vi "ClimbExecuteLogic.vi"(8 "error in (no error)":errorcluster, 9 "PullLS":bool, 10 "ReachLS":bool, 11 "SensorPosition":dbl) -> (0 "error out":errorcluster, 2 "ClimbStates":T1, 3 "MotorDemand":dbl)   [LabVIEW 2023]
doc: "Holds the \"insides\" for the elevator execution"
uses:
  <vilib>/Rock Robotics/WPI/ThirdParty/JAS_Junk/TrajLib/Trajectory_Library.lvlib
  ClimbGlobal.vi
  ClimbStates.ctl
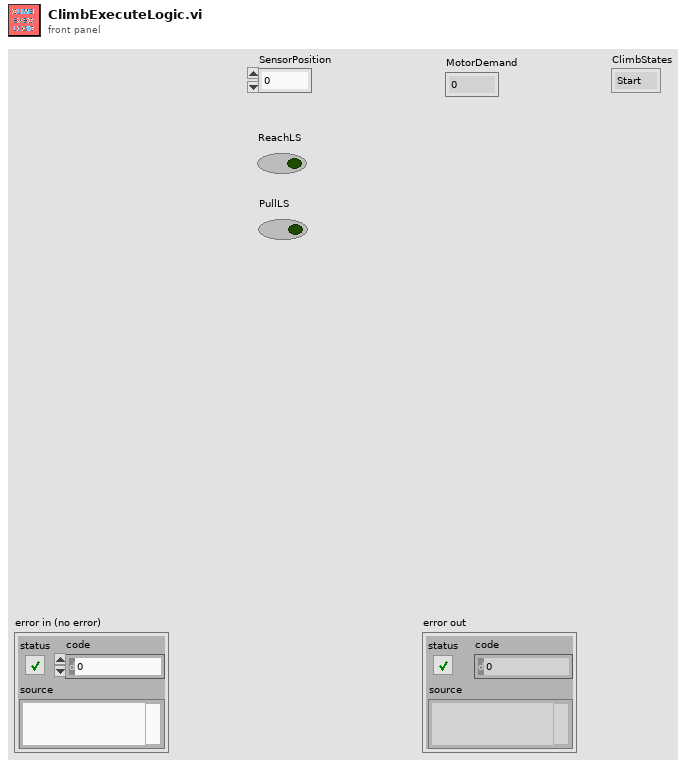
[diagram p1: front panel]
types:
  T1 = typedef "ClimbStates.ctl" = enum16{"Start", "WaitForCommands", "ClimbRest", "ClimbReach", "ClimbPull", "ClimbHang"}
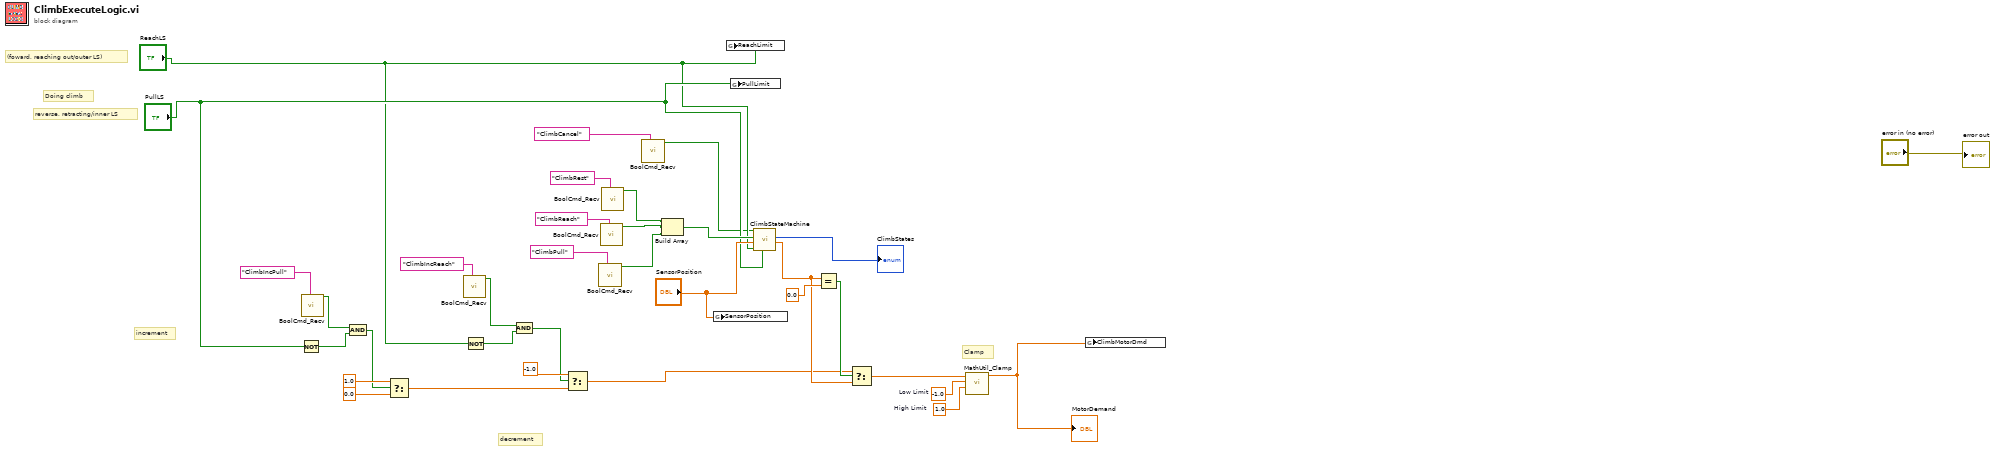
[diagram p0: block diagram]
diagram:
  w30 = 1.0  # High Limit
  w29 = -1.0  # Low Limit
  # "Doing climb"
  # "reverse, retracting/inner LS"
  # "(foward, reaching out/outer LS)"
  # "Clamp"
  # "increment"
  # "decrement"
  n1 = Not(x="PullLS") -> (.not. x?=w13:bool)
  n2 = call <vilib>:"BoolCmd_Recv.vi"("Command Name"="ClimbIncPull") -> ("New Request"=w1:bool)  [unwired: 9 in, 1 out]
  n3 = And(x=w1, y=w13) -> (x .and. y?=w12:bool)
  n4 = Select(t=1.0, s=w12, f=0.0) -> (s? t:f=w24:dbl)
  n5 = call <vilib>:"BoolCmd_Recv.vi"("Command Name"="ClimbIncReach") -> ("New Request"=w2:bool)  [unwired: 9 in, 1 out]
  n6 = Not(x="ReachLS") -> (.not. x?=w10:bool)
  n7 = And(x=w2, y=w10) -> (x .and. y?=w11:bool)
  n8 = Select(t=-1.0, s=w11, f=w24) -> (s? t:f=w22:dbl)
  n9 = call <vilib>:"BoolCmd_Recv.vi"("Command Name"="ClimbPull") -> ("New Request"=w3:bool)  [unwired: 9 in, 1 out]
  n10 = call <vilib>:"BoolCmd_Recv.vi"("Command Name"="ClimbReach") -> ("New Request"=w4:bool)  [unwired: 9 in, 1 out]
  n11 = call <vilib>:"BoolCmd_Recv.vi"("Command Name"="ClimbRest") -> ("New Request"=w5:bool)  [unwired: 9 in, 1 out]
  n12 = call <vilib>:"BoolCmd_Recv.vi"("Command Name"="ClimbCancel") -> ("New Request"=w6:bool)  [unwired: 9 in, 1 out]
  n13 = Build Array(w5, w4, w3) -> (w14:bool[])
  n14 = global write "ClimbGlobal.vi" "SensorPosition"("SensorPosition") -> ()
  n15 = global write "ClimbGlobal.vi" "ReachLimit"("ReachLS") -> ()
  n16 = global write "ClimbGlobal.vi" "PullLimit"("PullLS") -> ()
  n17 = call "ClimbStateMachine.vi"("PullLS"="PullLS", "ReachLS"="ReachLS", "ClimbEncoder"="SensorPosition", "Array"=w14, "Cancel"=w6) -> ("MotorOutput"=w31:dbl, "ClimbStates"=→"ClimbStates":T1)  [unwired: 5 in]
  n18 = Equal?(x=w31, y=0.0) -> (x = y?=w32:bool)
  n19 = Select(t=w22, s=w32, f=w31) -> (s? t:f=w27:dbl)
  n20 = call <vilib>:"MathUtil_Clamp.vi"("High Limit"=w30, "Low Limit"=w29, "Value"=w27) -> ("Result"=w28:dbl)  [unwired: 8 in]
  "MotorDemand" <- w28
  n21 = global write "ClimbGlobal.vi" "ClimbMotorDmd"(w28) -> ()
  "error out" <- "error in (no error)"
